vi "Main.vi"() -> (0 "error out":errorcluster, 3 "Weather Stations Data":T1)   [LabVIEW 2020, in "Netatmo-WeatherStation.lvlib"]
uses:
  Netatmo-WeatherStation.lvlib
  TypeDefs/body.ctl
  TypeDefs/devices.items.ctl
  TypeDefs/place.ctl
  TypeDefs/devices.dashboard_data.ctl
  TypeDefs/modules.items.ctl
  TypeDefs/modules.dashboard_data.ctl
  TypeDefs/user.ctl
  TypeDefs/administrative.ctl
  a4aeac39-dd97-49b2-b57e-7c1d20301938.vi
  <vilib>/JDP Science/JSONtext/Find Item.vi
  <vilib>/JDP Science/JSONtext/String Subset.vi
  subVIs/globals.vi
  <vilib>/JDP Science/JSONtext/Parsing/Parse Full Path or Item Name.vi
  <vilib>/JDP Science/JSONtext/Next JSON Value.vi
  <vilib>/JDP Science/JSONtext/support/Error Cluster From Code.vi
  <vilib>/JDP Science/JSONtext/Offset/Find Item Locations by Path.vi
  <vilib>/JDP Science/JSONtext/JSON text to Variant.vi
panel:
  out "Weather Stations Data (JSON)":string
  out "access token":string caption="<JSON>Item"
  out "state mismatch":bool
  # "DO NOT FORGET TO START and stop THE WEB SERVICE manually!\n\nRight click on “OAuth” in the Project Window and select Application Web Server>>Start (Debug Server) to start the web service."
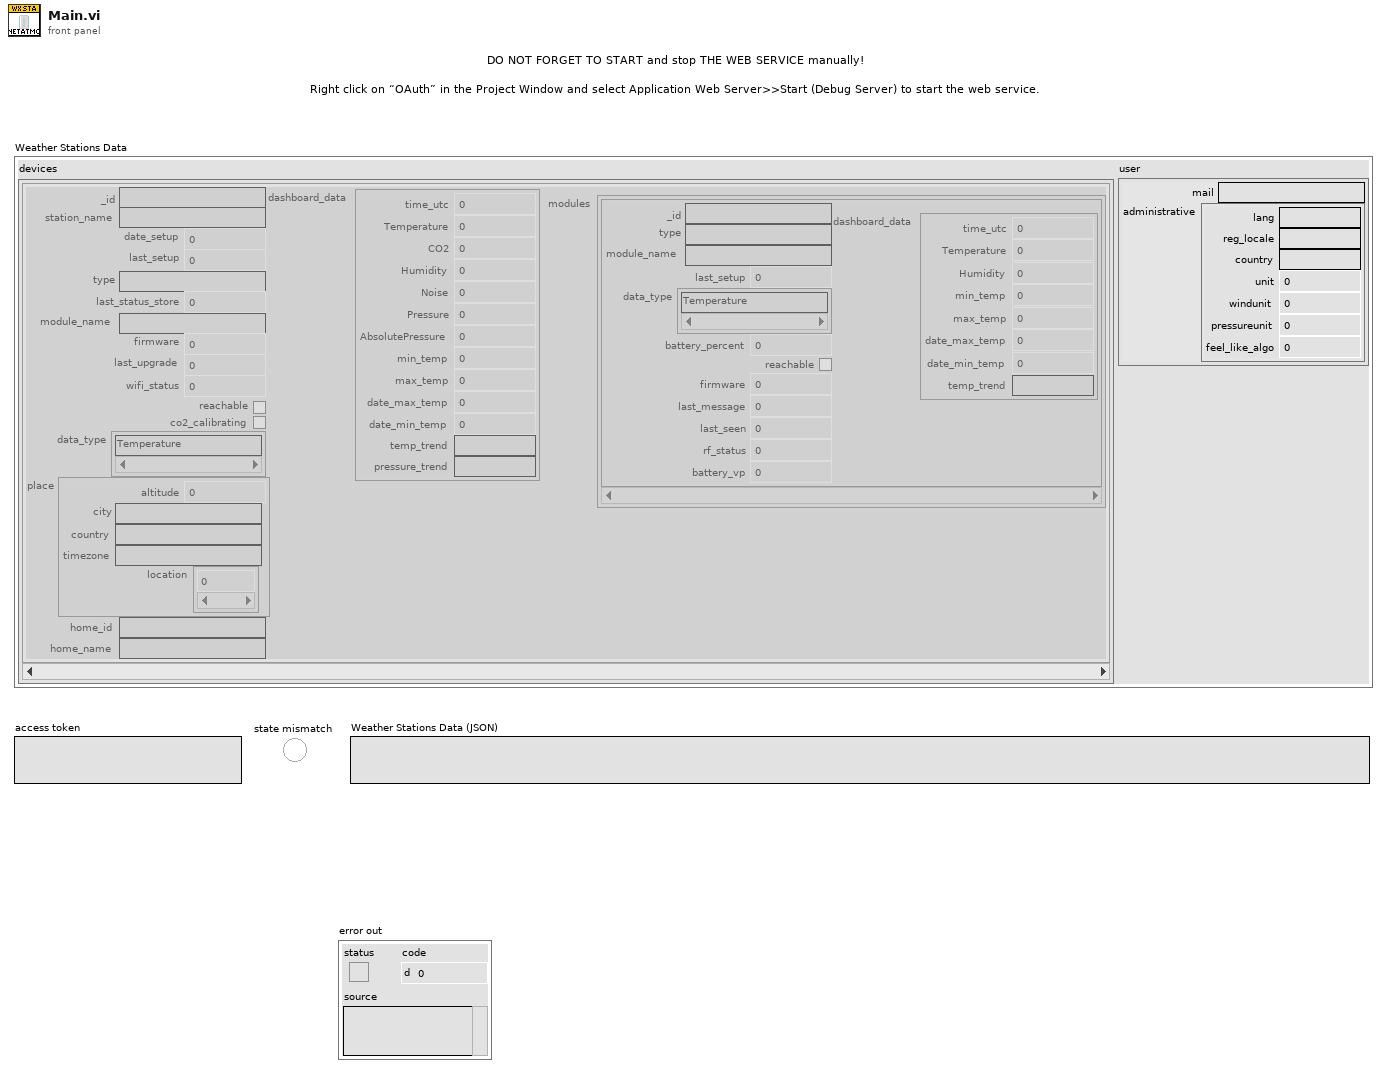
[diagram p1: front panel]
types:
  T1 = typedef "Netatmo-WeatherStation.lvlib/body.ctl" = cluster{"devices":T2[], "user":T7}
  T2 = typedef "Netatmo-WeatherStation.lvlib/devices.items.ctl" = cluster{"_id":string, "station_name":string, "date_setup":dbl, "last_setup":dbl, "type":string, "last_status_store":dbl, "module_name":string, "firmware":dbl, "last_upgrade":dbl, "wifi_status":dbl, "reachable":bool, "co2_calibrating":bool, "data_type":string[], "place":T3, "home_id":string, "home_name":string, "dashboard_data":T4, "modules":T5[]}
  T3 = typedef "Netatmo-WeatherStation.lvlib/place.ctl" = cluster{"altitude":dbl, "city":string, "country":string, "timezone":string, "location":dbl[]}
  T4 = typedef "Netatmo-WeatherStation.lvlib/devices.dashboard_data.ctl" = cluster{"time_utc":dbl, "Temperature":dbl, "CO2":dbl, "Humidity":dbl, "Noise":dbl, "Pressure":dbl, "AbsolutePressure":dbl, "min_temp":dbl, "max_temp":dbl, "date_max_temp":dbl, "date_min_temp":dbl, "temp_trend":string, "pressure_trend":string}
  T5 = typedef "Netatmo-WeatherStation.lvlib/modules.items.ctl" = cluster{"_id":string, "type":string, "module_name":string, "last_setup":dbl, "data_type":string[], "battery_percent":dbl, "reachable":bool, "firmware":dbl, "last_message":dbl, "last_seen":dbl, "rf_status":dbl, "battery_vp":dbl, "dashboard_data":T6}
  T6 = typedef "Netatmo-WeatherStation.lvlib/modules.dashboard_data.ctl" = cluster{"time_utc":dbl, "Temperature":dbl, "Humidity":dbl, "min_temp":dbl, "max_temp":dbl, "date_max_temp":dbl, "date_min_temp":dbl, "temp_trend":string}
  T7 = typedef "Netatmo-WeatherStation.lvlib/user.ctl" = cluster{"mail":string, "administrative":T8}
  T8 = typedef "Netatmo-WeatherStation.lvlib/administrative.ctl" = cluster{"lang":string, "reg_locale":string, "country":string, "unit":dbl, "windunit":dbl, "pressureunit":dbl, "feel_like_algo":dbl}
  T9 = cluster{"Redirect Data":refnum<user-event>, "Redirect Error":refnum<user-event>}
  T10 = cluster{"body":T1, "status":string, "time_exec":dbl, "time_server":dbl}
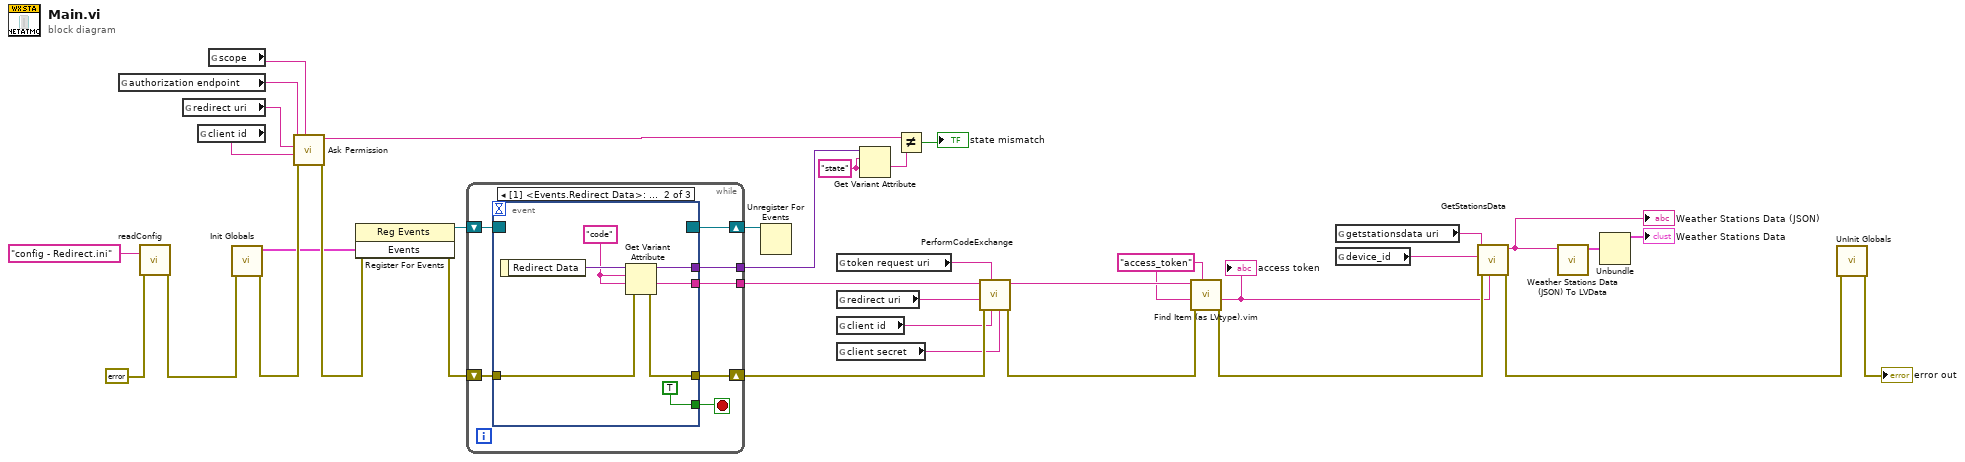
[diagram p0: block diagram]
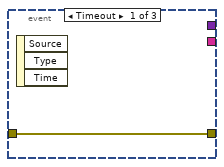
[diagram p2: hidden frame]
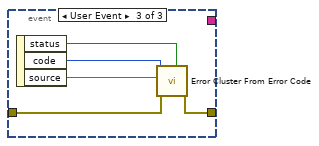
[diagram p3: hidden frame]
diagram:
  w13 = "state" ("key")
  w29 = "access_token" ("key")
  n1 = global read "globals.vi" "authorization endpoint"() -> (w21:string)
  n2 = call "readConfig.vi"("error in (no error)"=errorcluster {"status"=FALSE, "code"=0, "source"=""} ("error in"), "Config File Name"="config - Redirect.ini") -> ("error out"=w2:errorcluster)  [unwired: 9 in]
  n3 = global read "globals.vi" "redirect uri"() -> (w20:string)
  n4 = global read "globals.vi" "client id"() -> (w18:string)
  n5 = global read "globals.vi" "scope"() -> (w19:string)
  n6 = call "Init Globals.vi"("error in"=w2) -> ("error out"=w33:errorcluster, "Events"=w22:T9)  [unwired: 9 in]
  n7 = call "Ask Permission.vi"("scope"=w19, "error in (no error)"=w33, "client id"=w18, "redirect uri"=w20, "authorization endpoint"=w21) -> ("error out"=w36:errorcluster, "original state"=w35:string)  [unwired: 5 in]
  n8 = register-events(error in=w36, w22) -> (reference out=w28:refnum<event-registration>, error out=w27:errorcluster)  [unwired: 1 in]
  n9 = while {
    shift-right: [w41] -> w25
    shift-left: w27 -> [w42]
    shift-right: [w40] -> w26
    shift-left: w28 -> [w43]
    tunnel: [w38] -> w23
    tunnel: [w37] -> w24
    stop <- w39 stop-if-true
    n10 = event shown="[1] <Events.Redirect Data>: User Event" {
      selector: w43 -> [_ _ _]
      dyn-events: [_ _ _] -> w40
      timeout: _ -> [_ _ _]
      tunnel: w42 -> [w44 w46 w54]
      tunnel: [w44 w45 w53] -> w41
      tunnel: [_ TRUE _] -> w39
      tunnel: [_ w48 _] -> w38
      tunnel: [_ w47 _] -> w37
      event Timeout {
        n11 = event-data() -> ()  [unwired: 1 in, 3 out]
      }
      event User Event {
        w49 = "code" ("key")
        n12 = event-data() -> ("Redirect Data"=w50:variant)  [unwired: 1 in]
        n13 = Get Variant Attribute(Variant=w50, name=w49, default value (empty Variant)=w49, error in=w46) -> (duplicate Variant=w47:variant, value=w48:string, error out=w45:errorcluster)  [unwired: 1 out]
      }
      event User Event {
        n14 = event-data() -> ("status"=w52:bool, "code"=w55:i32, "source"=w56:string)  [unwired: 1 in]
        n15 = call <vilib>:"Error Cluster From Error Code.vi"("is warning? (False)"=w52, "error in (no error)"=w54, "error message (\"\")"=w56, "error code (0)"=w55) -> ("error out"=w53:errorcluster)  [unwired: 5 in]
      }
    }
  }
  n16 = Unregister For Events(event registration refnum=w26) -> ()  [unwired: 1 in, 1 out]
  n17 = global read "globals.vi" "token request uri"() -> (w14:string)
  n18 = global read "globals.vi" "redirect uri"() -> (w15:string)
  n19 = global read "globals.vi" "client id"() -> (w17:string)
  n20 = global read "globals.vi" "client secret"() -> (w16:string)
  n21 = Get Variant Attribute(Variant=w24, name=w13, default value (empty Variant)=w13) -> (value=w34:string)  [unwired: 1 in, 3 out]
  n22 = Not Equal?(x=w35, y=w34) -> (x != y?=→"state mismatch":bool)
  n23 = call "PerformCodeExchange.vi"("client secret"=w16, "client id"=w17, "token request uri"=w14, "error in (no error)"=w25, "redirect uri"=w15, "code"=w23) -> ("error out"=w30:errorcluster, "token response (JSON)"=w31:string)  [unwired: 4 in]
  n24 = call "Find Item (as LVtype).vim"("$Path or Item Name"=w29, "error in (no error)"=w30, "Data Type and Default Value"=w29, "JSON"=w31) -> ("error out"=w12:errorcluster, "Data"=w11:string)  [unwired: 4 in, 2 out]
  "access token" <- w11
  n25 = global read "globals.vi" "getstationsdata uri"() -> (w10:string)
  n26 = global read "globals.vi" "device_id"() -> (w9:string)
  n27 = call "GetStationsData.vi"("access token"=w11, "error in (no error)"=w12, "device_id"=w9, "token request uri"=w10) -> ("error out"=w8:errorcluster, "Weather Stations Data (JSON)"=w6:string)  [unwired: 6 in]
  "Weather Stations Data (JSON)" <- w6
  n28 = call "Weather Stations Data (JSON) To LVData.vi"("Weather Stations Data (JSON)"=w6) -> ("Data"=w5:T10)  [unwired: 9 in, 1 out]
  n29 = Unbundle(w5) -> ("body"=→"Weather Stations Data":T1)  [unwired: 3 out]
  n30 = call "UnInit Globals.vi"("error in"=w8) -> ("error out"=→"error out":errorcluster)  [unwired: 10 in]
